vi "Lab Panel V5.10.vi"() -> ()   [LabVIEW 2013] (continued)
                            n848 = local write "data file error"(w1525) -> ()
                          }
                        }
                        n849 = Bundle(cluster=w1522, "STATUS"="STOP") -> (w1520:T4)  [unwired: 2 in]
                        n850 = local write "DISP LAB04-1"(w1520) -> ()
                      }
                    }
                  }
                  frame True {
                    n851 = local read "SIG LAB04-1"() -> (w1529:T2)
                    n852 = stacked-sequence {
                      seq-local: [w1540 _] -> [_ w1544]
                      tunnel: w1538 -> [_ w1554]
                      tunnel: w1537 -> [_ w1553]
                      tunnel: w1536 -> [_ w1552]
                      tunnel: w1535 -> [_ w1551]
                      tunnel: w1534 -> [_ w1550]
                      tunnel: [_ w1549] -> w1533
                      tunnel: w1532 -> [_ w1548]
                      tunnel: w1531 -> [_ w1547]
                      tunnel: w1530 -> [_ w1546]
                      tunnel: w1529 -> [w1539 w1545]
                      tunnel: w1528 -> [_ w1543]
                      frame #0 {
                        n853 = Unbundle(w1539) -> ("AMPS"=w1542:dbl)  [unwired: 4 out]
                        n854 = call "Check For Amps on v1.vi"("ID"="LAB04-1", "amps"=w1542) -> ("amps"=w1540:bool)  [unwired: 9 in]
                      }
                      frame #1 {
                        n855 = case shown="True" w1544 {
                          tunnel: w1554 -> [_ w1567]
                          tunnel: w1553 -> [_ w1566]
                          tunnel: w1552 -> [_ w1565]
                          tunnel: w1551 -> [_ w1564]
                          tunnel: w1550 -> [_ w1563]
                          tunnel: [errorcluster {"status"=FALSE, "code"=0, "source"=""} ("error out") w1562] -> w1549
                          tunnel: w1548 -> [_ w1561]
                          tunnel: w1547 -> [_ w1560]
                          tunnel: w1546 -> [_ w1559]
                          tunnel: w1545 -> [_ w1558]
                          tunnel: w1543 -> [_ w1557]
                          frame False {
                            w1555 = FALSE
                            n856 = local write "RUN LAB04-1"(w1555) -> ()
                            n857 = local write "run lab04-1"(w1555) -> ()
                          }
                          frame True {
                            n858 = stacked-sequence {
                              seq-local: [w1568 _ _ _ _] -> [_ w1592 _ _ _]
                              tunnel: w1567 -> [w1573 _ _ _ _]
                              tunnel: w1566 -> [w1569 _ _ _ _]
                              tunnel: w1565 -> [w1583 _ _ _ _]
                              tunnel: w1564 -> [w1576 _ _ _ _]
                              tunnel: w1563 -> [w1571 _ _ _ _]
                              tunnel: [_ w1587 _ _ _] -> w1562
                              tunnel: w1561 -> [_ _ _ w1613 _]
                              tunnel: w1560 -> [_ _ _ w1612 _]
                              tunnel: w1559 -> [_ _ _ w1611 _]
                              tunnel: w1558 -> [_ _ _ _ _]
                              tunnel: w1557 -> [_ _ _ _ w1627]
                              frame #0 {
                                w1570 = "\\"
                                n859 = local read "SET LAB04-1"() -> (w1578:T5)
                                n860 = case shown="\"CYCLE TEST\"" w1583 {
                                tunnel: ["L04-1-CHART TEST-" "L04-1-CYCLE TEST-" "L04-1-T-RISE TEST-"] -> w1579
                                frame "CHART TEST", Default {
                                }
                                frame "CYCLE TEST" {
                                }
                                frame "T-RISE TEST" {
                                }
                                }
                                n861 = Unbundle(w1578) -> ("DESCRIPTION"=w1577:string)  [unwired: 4 out]
                                n862 = Concatenate Strings(w1573, "\\", w1571, w1570, w1569, w1570) -> (w1580:string)
                                n863 = String To Path(string=w1580) -> (path=w1582:path)
                                n864 = Concatenate Strings(w1580, w1579, w1577, "-", w1576, ".tdms") -> (w1568:string)
                                n865 = Create Folder(path (use dialog)=w1582) -> (error out=w1581:errorcluster)  [unwired: 2 in, 2 out]
                                n866 = global write "Global 1.vi" "LAB04-1 FILE"(w1568) -> ()
                                n867 = call <vilib>:"Clear Errors.vi"("error in (no error)"=w1581) -> ()  [unwired: 6 in, 1 out]
                              }
                              frame #1 {
                                (unwired) FALSE
                                n868 = String To Path(string=w1592) -> (path=w1588:path)
                                n869 = TDMS Open(6:FALSE, 10:T20."create or replace" ("operation (0:open)"), 11:w1588) -> (0:w1587:errorcluster, 3:→"TDMS LAB04-1":refnum<k34>)  [unwired: 4 in]
                              }
                              frame #2 {
                                n870 = local read "SET LAB04-1"() -> (w1598:T5)
                                n871 = local read "TDMS LAB04-1"() -> (w1609:refnum<k34>)
                                n872 = Build Array("Testers Name", "Description", "Set Test Cycles", "T-Rise minutes", "T-Rise Deg C") -> (w1599:string[])
                                n873 = Unbundle(w1598) -> ("NAME"=w1597:string, "DESCRIPTION"=w1596:string, "CYCLES"=w1595:dbl, "T-RISE mins"=w1594:dbl, "T-RISE deg C"=w1593:dbl)
                                n874 = Number To Decimal String(number=w1595) -> (decimal integer string=w1608:string)  [unwired: 1 in]
                                n875 = Number To Decimal String(number=w1594) -> (decimal integer string=w1607:string)  [unwired: 1 in]
                                n876 = Number To Decimal String(number=w1593) -> (decimal integer string=w1606:string)  [unwired: 1 in]
                                n877 = Build Array(w1597, w1596, w1608, w1607, w1606) -> (w1605:string[])
                                n878 = TDMS Set Properties(5:w1605, 7:w1599, 11:w1609) -> ()  [unwired: 3 in, 4 out]
                              }
                              frame #3 {
                                n879 = local read "DISP LAB04-1"() -> (w1614:T4)
                                n880 = Concatenate Strings("LAB04-1  ", w1613) -> (w1615:string)
                                n881 = Two Button Dialog(message=w1615, 1:w1611, 2:w1612) -> (T button?=w1617:bool)
                                n882 = case shown="True" w1617 {
                                tunnel: w1614 -> [w1624 w1625]
                                tunnel: [w1624 w1625] -> w1621
                                tunnel: [w1623 w1626] -> w1620
                                tunnel: [w1622 w1626] -> w1619
                                frame False {
                                n883 = Unbundle(w1624) -> ("CYCLE"=w1623:dbl, "MINS"=w1622:dbl)  [unwired: 1 out]
                                }
                                frame True {
                                w1626 = 0.0
                                }
                                }
                                n884 = Bundle(cluster=w1621, "CYCLE"=w1620, "MINS"=w1619, "STATUS"="RUN") -> (w1610:T4)
                                n885 = local write "DISP LAB04-1"(w1610) -> ()
                              }
                              frame #4 {
                                n886 = local read "TEMP START LAB04-1"() -> (w1629:cluster{"TL":dbl, "TN":dbl})
                                n887 = Bundle(cluster=w1629, "TL"=w1627, "TN"=w1627) -> (w1628:cluster{"TL":dbl, "TN":dbl})
                                n888 = local write "TEMP START LAB04-1"(w1628) -> ()
                              }
                            }
                          }
                        }
                      }
                    }
                  }
                }
              }
              event "RUN LAB04-2": Value Change {
                n889 = event-data() -> ("NewVal"=w1634:bool)  [unwired: 1 in, 5 out]
                n890 = local write "run lab04-2"(w1634) -> ()
                n891 = case shown="True" w1634 {
                  tunnel: w1640 -> [_ w1678]
                  tunnel: w1639 -> [_ w1677]
                  tunnel: w1637 -> [w1642 w1676]
                  tunnel: w1638 -> [_ w1675]
                  tunnel: w1636 -> [_ w1674]
                  tunnel: [w1641 w1673] -> w1635
                  tunnel: w1633 -> [_ w1672]
                  tunnel: w1632 -> [_ w1671]
                  tunnel: w1631 -> [_ w1670]
                  tunnel: w1630 -> [_ w1668]
                  frame False {
                    # "stop test"
                    n892 = stacked-sequence {
                      tunnel: w1642 -> [w1651 _]
                      tunnel: [w1643 _] -> w1641
                      frame #0 {
                        n893 = local read "DISP LAB04-2"() -> (w1650:T4)
                        n894 = Unbundle(w1650) -> ("CYCLE"=w1648:dbl, "MINS"=w1649:dbl)  [unwired: 1 out]
                        n895 = case shown="\"CYCLE TEST\"" w1651 {
                          tunnel: w1649 -> [_ _ w1658]
                          tunnel: w1648 -> [w1656 w1657 _]
                          tunnel: [w1656 w1657 w1658] -> w1647
                          frame "CHART TEST", Default {
                          }
                          frame "CYCLE TEST" {
                          }
                          frame "T-RISE TEST" {
                          }
                        }
                        n896 = local read "TDMS LAB04-2"() -> (w1655:refnum<k34>)
                        n897 = Build Array("STOPPED") -> (w1652:string[])
                        n898 = Build Array(w1647) -> (w1646:dbl[])
                        n899 = TDMS Write(0:w1655, 5:"TEST RESULT", 7:w1652, 9:w1646) -> (4:w1644:refnum<k34>, 15:w1645:errorcluster)  [unwired: 2 in, 2 out]
                        n900 = TDMS Close(8:w1645, 11:w1644) -> (0:w1643:errorcluster)  [unwired: 1 out]
                      }
                      frame #1 {
                        n901 = local read "DISP LAB04-2"() -> (w1662:T4)
                        n902 = stacked-sequence {
                          tunnel: "LAB04-2" -> [w1664 w1666]
                          frame #0 {
                            n903 = call "sub vi - defrag tdms v1.vi"("panel id"=w1664) -> ("error out"=w1663:errorcluster)  [unwired: 10 in]
                            n904 = local write "data file error"(w1663) -> ()
                          }
                          frame #1 {
                            n905 = call "Save data file (stop) v3.vi"("panel id"=w1666) -> ("network file save error"=w1665:errorcluster)  [unwired: 9 in, 1 out]
                            n906 = local write "RESULT LAB04-2"(FALSE) -> ()
                            n907 = local write "data file error"(w1665) -> ()
                          }
                        }
                        n908 = Bundle(cluster=w1662, "STATUS"="STOP") -> (w1660:T4)  [unwired: 2 in]
                        n909 = local write "DISP LAB04-2"(w1660) -> ()
                      }
                    }
                  }
                  frame True {
                    n910 = local read "SIG LAB04-2"() -> (w1669:T2)
                    n911 = stacked-sequence {
                      seq-local: [w1680 _] -> [_ w1684]
                      tunnel: w1678 -> [_ w1694]
                      tunnel: w1677 -> [_ w1693]
                      tunnel: w1676 -> [_ w1692]
                      tunnel: w1675 -> [_ w1691]
                      tunnel: w1674 -> [_ w1690]
                      tunnel: [_ w1689] -> w1673
                      tunnel: w1672 -> [_ w1688]
                      tunnel: w1671 -> [_ w1687]
                      tunnel: w1670 -> [_ w1686]
                      tunnel: w1669 -> [w1679 w1685]
                      tunnel: w1668 -> [_ w1683]
                      frame #0 {
                        n912 = Unbundle(w1679) -> ("AMPS"=w1682:dbl)  [unwired: 4 out]
                        n913 = call "Check For Amps on v1.vi"("ID"="LAB04-2", "amps"=w1682) -> ("amps"=w1680:bool)  [unwired: 9 in]
                      }
                      frame #1 {
                        n914 = case shown="True" w1684 {
                          tunnel: w1694 -> [_ w1707]
                          tunnel: w1693 -> [_ w1706]
                          tunnel: w1692 -> [_ w1705]
                          tunnel: w1691 -> [_ w1704]
                          tunnel: w1690 -> [_ w1703]
                          tunnel: [errorcluster {"status"=FALSE, "code"=0, "source"=""} ("error out") w1702] -> w1689
                          tunnel: w1688 -> [_ w1701]
                          tunnel: w1687 -> [_ w1700]
                          tunnel: w1686 -> [_ w1699]
                          tunnel: w1685 -> [_ w1698]
                          tunnel: w1683 -> [_ w1697]
                          frame False {
                            w1695 = FALSE
                            n915 = local write "RUN LAB04-2"(w1695) -> ()
                            n916 = local write "run lab04-2"(w1695) -> ()
                          }
                          frame True {
                            n917 = stacked-sequence {
                              seq-local: [w1708 _ _ _ _] -> [_ w1732 _ _ _]
                              tunnel: w1707 -> [w1713 _ _ _ _]
                              tunnel: w1706 -> [w1709 _ _ _ _]
                              tunnel: w1705 -> [w1723 _ _ _ _]
                              tunnel: w1704 -> [w1716 _ _ _ _]
                              tunnel: w1703 -> [w1711 _ _ _ _]
                              tunnel: [_ w1727 _ _ _] -> w1702
                              tunnel: w1701 -> [_ _ _ w1753 _]
                              tunnel: w1700 -> [_ _ _ w1752 _]
                              tunnel: w1699 -> [_ _ _ w1751 _]
                              tunnel: w1698 -> [_ _ _ _ _]
                              tunnel: w1697 -> [_ _ _ _ w1767]
                              frame #0 {
                                w1710 = "\\"
                                n918 = local read "SET LAB04-2"() -> (w1718:T5)
                                n919 = case shown="\"CHART TEST\", Default" w1723 {
                                tunnel: ["L04-2-CHART TEST-" "L04-2-CYCLE TEST-" "L04-2-T-RISE TEST-"] -> w1719
                                frame "CHART TEST", Default {
                                }
                                frame "CYCLE TEST" {
                                }
                                frame "T-RISE TEST" {
                                }
                                }
                                n920 = Unbundle(w1718) -> ("DESCRIPTION"=w1717:string)  [unwired: 4 out]
                                n921 = Concatenate Strings(w1713, "\\", w1711, w1710, w1709, w1710) -> (w1720:string)
                                n922 = String To Path(string=w1720) -> (path=w1722:path)
                                n923 = Concatenate Strings(w1720, w1719, w1717, "-", w1716, ".tdms") -> (w1708:string)
                                n924 = Create Folder(path (use dialog)=w1722) -> (error out=w1721:errorcluster)  [unwired: 2 in, 2 out]
                                n925 = global write "Global 1.vi" "LAB04-2 FILE"(w1708) -> ()
                                n926 = call <vilib>:"Clear Errors.vi"("error in (no error)"=w1721) -> ()  [unwired: 6 in, 1 out]
                              }
                              frame #1 {
                                (unwired) FALSE
                                n927 = String To Path(string=w1732) -> (path=w1728:path)
                                n928 = TDMS Open(6:FALSE, 10:T20."create or replace" ("operation (0:open)"), 11:w1728) -> (0:w1727:errorcluster, 3:→"TDMS LAB04-2":refnum<k34>)  [unwired: 4 in]
                              }
                              frame #2 {
                                n929 = local read "SET LAB04-2"() -> (w1738:T5)
                                n930 = local read "TDMS LAB04-2"() -> (w1749:refnum<k34>)
                                n931 = Build Array("Testers Name", "Description", "Set Test Cycles", "T-Rise minutes", "T-Rise Deg C") -> (w1739:string[])
                                n932 = Unbundle(w1738) -> ("NAME"=w1737:string, "DESCRIPTION"=w1736:string, "CYCLES"=w1735:dbl, "T-RISE mins"=w1734:dbl, "T-RISE deg C"=w1733:dbl)
                                n933 = Number To Decimal String(number=w1735) -> (decimal integer string=w1748:string)  [unwired: 1 in]
                                n934 = Number To Decimal String(number=w1734) -> (decimal integer string=w1747:string)  [unwired: 1 in]
                                n935 = Number To Decimal String(number=w1733) -> (decimal integer string=w1746:string)  [unwired: 1 in]
                                n936 = Build Array(w1737, w1736, w1748, w1747, w1746) -> (w1745:string[])
                                n937 = TDMS Set Properties(5:w1745, 7:w1739, 11:w1749) -> ()  [unwired: 3 in, 4 out]
                              }
                              frame #3 {
                                n938 = local read "DISP LAB04-2"() -> (w1754:T4)
                                n939 = Concatenate Strings("LAB04-2 ", w1753) -> (w1755:string)
                                n940 = Two Button Dialog(message=w1755, 1:w1751, 2:w1752) -> (T button?=w1757:bool)
                                n941 = case shown="True" w1757 {
                                tunnel: w1754 -> [w1764 w1765]
                                tunnel: [w1764 w1765] -> w1761
                                tunnel: [w1763 w1766] -> w1760
                                tunnel: [w1762 w1766] -> w1759
                                frame False {
                                n942 = Unbundle(w1764) -> ("CYCLE"=w1763:dbl, "MINS"=w1762:dbl)  [unwired: 1 out]
                                }
                                frame True {
                                w1766 = 0.0
                                }
                                }
                                n943 = Bundle(cluster=w1761, "CYCLE"=w1760, "MINS"=w1759, "STATUS"="RUN") -> (w1750:T4)
                                n944 = local write "DISP LAB04-2"(w1750) -> ()
                              }
                              frame #4 {
                                n945 = local read "TEMP START LAB04-2"() -> (w1769:cluster{"TL":dbl, "TN":dbl})
                                n946 = Bundle(cluster=w1769, "TL"=w1767, "TN"=w1767) -> (w1768:cluster{"TL":dbl, "TN":dbl})
                                n947 = local write "TEMP START LAB04-2"(w1768) -> ()
                              }
                            }
                          }
                        }
                      }
                    }
                  }
                }
              }
              event "RUN LAB05-1": Value Change {
                n948 = event-data() -> ("NewVal"=w1774:bool)  [unwired: 1 in, 5 out]
                n949 = local write "run lab05-1"(w1774) -> ()
                n950 = case shown="True" w1774 {
                  tunnel: w1780 -> [_ w1818]
                  tunnel: w1779 -> [_ w1817]
                  tunnel: w1777 -> [w1782 w1816]
                  tunnel: w1778 -> [_ w1815]
                  tunnel: w1776 -> [_ w1814]
                  tunnel: [w1781 w1813] -> w1775
                  tunnel: w1773 -> [_ w1812]
                  tunnel: w1772 -> [_ w1811]
                  tunnel: w1771 -> [_ w1810]
                  tunnel: w1770 -> [_ w1808]
                  frame False {
                    # "stop test"
                    n951 = stacked-sequence {
                      tunnel: w1782 -> [w1791 _]
                      tunnel: [w1783 _] -> w1781
                      frame #0 {
                        n952 = local read "DISP LAB05-1"() -> (w1790:T4)
                        n953 = Unbundle(w1790) -> ("CYCLE"=w1788:dbl, "MINS"=w1789:dbl)  [unwired: 1 out]
                        n954 = case shown="\"CYCLE TEST\"" w1791 {
                          tunnel: w1789 -> [_ _ w1798]
                          tunnel: w1788 -> [w1796 w1797 _]
                          tunnel: [w1796 w1797 w1798] -> w1787
                          frame "CHART TEST", Default {
                          }
                          frame "CYCLE TEST" {
                          }
                          frame "T-RISE TEST" {
                          }
                        }
                        n955 = local read "TDMS LAB05-1"() -> (w1795:refnum<k34>)
                        n956 = Build Array("STOPPED") -> (w1792:string[])
                        n957 = Build Array(w1787) -> (w1786:dbl[])
                        n958 = TDMS Write(0:w1795, 5:"TEST RESULT", 7:w1792, 9:w1786) -> (4:w1784:refnum<k34>, 15:w1785:errorcluster)  [unwired: 2 in, 2 out]
                        n959 = TDMS Close(8:w1785, 11:w1784) -> (0:w1783:errorcluster)  [unwired: 1 out]
                      }
                      frame #1 {
                        n960 = local read "DISP LAB05-1"() -> (w1802:T4)
                        n961 = stacked-sequence {
                          tunnel: "LAB05-1" -> [w1804 w1806]
                          frame #0 {
                            n962 = call "sub vi - defrag tdms v1.vi"("panel id"=w1804) -> ("error out"=w1803:errorcluster)  [unwired: 10 in]
                            n963 = local write "data file error"(w1803) -> ()
                          }
                          frame #1 {
                            n964 = call "Save data file (stop) v3.vi"("panel id"=w1806) -> ("network file save error"=w1805:errorcluster)  [unwired: 9 in, 1 out]
                            n965 = local write "RESULT LAB05-1"(FALSE) -> ()
                            n966 = local write "data file error"(w1805) -> ()
                          }
                        }
                        n967 = Bundle(cluster=w1802, "STATUS"="STOP") -> (w1800:T4)  [unwired: 2 in]
                        n968 = local write "DISP LAB05-1"(w1800) -> ()
                      }
                    }
                  }
                  frame True {
                    n969 = local read "SIG LAB05-1"() -> (w1809:T2)
                    n970 = stacked-sequence {
                      seq-local: [w1820 _] -> [_ w1824]
                      tunnel: w1818 -> [_ w1834]
                      tunnel: w1817 -> [_ w1833]
                      tunnel: w1816 -> [_ w1832]
                      tunnel: w1815 -> [_ w1831]
                      tunnel: w1814 -> [_ w1830]
                      tunnel: [_ w1829] -> w1813
                      tunnel: w1812 -> [_ w1828]
                      tunnel: w1811 -> [_ w1827]
                      tunnel: w1810 -> [_ w1826]
                      tunnel: w1809 -> [w1819 w1825]
                      tunnel: w1808 -> [_ w1823]
                      frame #0 {
                        n971 = Unbundle(w1819) -> ("AMPS"=w1822:dbl)  [unwired: 4 out]
                        n972 = call "Check For Amps on v1.vi"("ID"="LAB05-1", "amps"=w1822) -> ("amps"=w1820:bool)  [unwired: 9 in]
                      }
                      frame #1 {
                        n973 = case shown="True" w1824 {
                          tunnel: w1834 -> [_ w1847]
                          tunnel: w1833 -> [_ w1846]
                          tunnel: w1832 -> [_ w1845]
                          tunnel: w1831 -> [_ w1844]
                          tunnel: w1830 -> [_ w1843]
                          tunnel: [errorcluster {"status"=FALSE, "code"=0, "source"=""} ("error out") w1842] -> w1829
                          tunnel: w1828 -> [_ w1841]
                          tunnel: w1827 -> [_ w1840]
                          tunnel: w1826 -> [_ w1839]
                          tunnel: w1825 -> [_ w1838]
                          tunnel: w1823 -> [_ w1837]
                          frame False {
                            w1835 = FALSE
                            n974 = local write "RUN LAB05-1"(w1835) -> ()
                            n975 = local write "run lab05-1"(w1835) -> ()
                          }
                          frame True {
                            n976 = stacked-sequence {
                              seq-local: [w1848 _ _ _ _] -> [_ w1872 _ _ _]
                              tunnel: w1847 -> [w1853 _ _ _ _]
                              tunnel: w1846 -> [w1849 _ _ _ _]
                              tunnel: w1845 -> [w1863 _ _ _ _]
                              tunnel: w1844 -> [w1856 _ _ _ _]
                              tunnel: w1843 -> [w1851 _ _ _ _]
                              tunnel: [_ w1867 _ _ _] -> w1842
                              tunnel: w1841 -> [_ _ _ w1892 _]
                              tunnel: w1840 -> [_ _ _ w1891 _]
                              tunnel: w1839 -> [_ _ _ w1890 _]
                              tunnel: w1838 -> [_ _ _ _ _]
                              tunnel: w1837 -> [_ _ _ _ w1907]
                              frame #0 {
                                w1850 = "\\"
                                n977 = local read "SET LAB05-1"() -> (w1858:T5)
                                n978 = case shown="\"CYCLE TEST\"" w1863 {
                                tunnel: ["L05-1-CHART TEST-" "L05-1-CYCLE TEST-" "L05-1-T-RISE TEST-"] -> w1859
                                frame "CHART TEST", Default {
                                }
                                frame "CYCLE TEST" {
                                }
                                frame "T-RISE TEST" {
                                }
                                }
                                n979 = Unbundle(w1858) -> ("DESCRIPTION"=w1857:string)  [unwired: 4 out]
                                n980 = Concatenate Strings(w1853, "\\", w1851, w1850, w1849, w1850) -> (w1860:string)
                                n981 = String To Path(string=w1860) -> (path=w1862:path)
                                n982 = Concatenate Strings(w1860, w1859, w1857, "-", w1856, ".tdms") -> (w1848:string)
                                n983 = Create Folder(path (use dialog)=w1862) -> (error out=w1861:errorcluster)  [unwired: 2 in, 2 out]
                                n984 = global write "Global 1.vi" "LAB05-1 FILE"(w1848) -> ()
                                n985 = call <vilib>:"Clear Errors.vi"("error in (no error)"=w1861) -> ()  [unwired: 6 in, 1 out]
                              }
                              frame #1 {
                                (unwired) FALSE
                                n986 = String To Path(string=w1872) -> (path=w1868:path)
                                n987 = TDMS Open(6:FALSE, 10:T20."create or replace" ("operation (0:open)"), 11:w1868) -> (0:w1867:errorcluster, 3:→"TDMS LAB05-1":refnum<k34>)  [unwired: 4 in]
                              }
                              frame #2 {
                                n988 = local read "SET LAB05-1"() -> (w1878:T5)
                                n989 = local read "TDMS LAB05-1"() -> (w1889:refnum<k34>)
                                n990 = Build Array("Testers Name", "Description", "Set Test Cycles", "T-Rise minutes", "T-Rise Deg C") -> (w1879:string[])
                                n991 = Unbundle(w1878) -> ("NAME"=w1877:string, "DESCRIPTION"=w1876:string, "CYCLES"=w1875:dbl, "T-RISE mins"=w1874:dbl, "T-RISE deg C"=w1873:dbl)
                                n992 = Number To Decimal String(number=w1875) -> (decimal integer string=w1888:string)  [unwired: 1 in]
                                n993 = Number To Decimal String(number=w1874) -> (decimal integer string=w1887:string)  [unwired: 1 in]
                                n994 = Number To Decimal String(number=w1873) -> (decimal integer string=w1886:string)  [unwired: 1 in]
                                n995 = Build Array(w1877, w1876, w1888, w1887, w1886) -> (w1885:string[])
                                n996 = TDMS Set Properties(5:w1885, 7:w1879, 11:w1889) -> ()  [unwired: 3 in, 4 out]
                              }
                              frame #3 {
                                n997 = local read "DISP LAB05-1"() -> (w1894:T4)
                                n998 = Concatenate Strings("LAB05-1  ", w1892) -> (w1895:string)
                                n999 = Two Button Dialog(message=w1895, 1:w1890, 2:w1891) -> (T button?=w1897:bool)
                                n1000 = case shown="True" w1897 {
                                tunnel: w1894 -> [w1904 w1905]
                                tunnel: [w1904 w1905] -> w1901
                                tunnel: [w1903 w1906] -> w1900
                                tunnel: [w1902 w1906] -> w1899
                                frame False {
                                n1001 = Unbundle(w1904) -> ("CYCLE"=w1903:dbl, "MINS"=w1902:dbl)  [unwired: 1 out]
                                }
                                frame True {
                                w1906 = 0.0
                                }
                                }
                                n1002 = Bundle(cluster=w1901, "CYCLE"=w1900, "MINS"=w1899, "STATUS"="RUN") -> (w1893:T4)
                                n1003 = local write "DISP LAB05-1"(w1893) -> ()
                              }
                              frame #4 {
                                n1004 = local read "TEMP START LAB05-1"() -> (w1909:cluster{"TL":dbl, "TN":dbl})
                                n1005 = Bundle(cluster=w1909, "TL"=w1907, "TN"=w1907) -> (w1908:cluster{"TL":dbl, "TN":dbl})
                                n1006 = local write "TEMP START LAB05-1"(w1908) -> ()
                              }
                            }
                          }
                        }
                      }
                    }
                  }
                }
              }
              event "RUN LAB05-2": Value Change {
                n1007 = event-data() -> ("NewVal"=w1915:bool)  [unwired: 1 in, 5 out]
                n1008 = local read "SIG LAB05-2"() -> (w1911:T2)
                n1009 = case shown="True" w1915 {
                  tunnel: w1921 -> [_ w1959]
                  tunnel: w1920 -> [_ w1958]
                  tunnel: w1918 -> [w1923 w1957]
                  tunnel: w1919 -> [_ w1956]
                  tunnel: w1917 -> [_ w1955]
                  tunnel: [w1922 w1954] -> w1916
                  tunnel: w1914 -> [_ w1953]
                  tunnel: w1913 -> [_ w1952]
                  tunnel: w1912 -> [_ w1951]
                  tunnel: w1911 -> [_ w1950]
                  tunnel: w1910 -> [_ w1949]
                  frame False {
                    # "stop test"
                    n1010 = stacked-sequence {
                      tunnel: w1923 -> [w1932 _]
                      tunnel: [w1924 _] -> w1922
                      frame #0 {
                        n1011 = local read "DISP LAB05-2"() -> (w1931:T4)
                        n1012 = Unbundle(w1931) -> ("CYCLE"=w1929:dbl, "MINS"=w1930:dbl)  [unwired: 1 out]
                        n1013 = case shown="\"CYCLE TEST\"" w1932 {
                          tunnel: w1930 -> [_ _ w1939]
                          tunnel: w1929 -> [w1937 w1938 _]
                          tunnel: [w1937 w1938 w1939] -> w1928
                          frame "CHART TEST", Default {
                          }
                          frame "CYCLE TEST" {
                          }
                          frame "T-RISE TEST" {
                          }
                        }
                        n1014 = local read "TDMS LAB05-2"() -> (w1936:refnum<k34>)
                        n1015 = Build Array("STOPPED") -> (w1933:string[])
                        n1016 = Build Array(w1928) -> (w1927:dbl[])
                        n1017 = TDMS Write(0:w1936, 5:"TEST RESULT", 7:w1933, 9:w1927) -> (4:w1925:refnum<k34>, 15:w1926:errorcluster)  [unwired: 2 in, 2 out]
                        n1018 = TDMS Close(8:w1926, 11:w1925) -> (0:w1924:errorcluster)  [unwired: 1 out]
                      }
                      frame #1 {
                        n1019 = local read "DISP LAB05-2"() -> (w1943:T4)
                        n1020 = stacked-sequence {
                          tunnel: "LAB05-2" -> [w1945 w1947]
                          frame #0 {
                            n1021 = call "sub vi - defrag tdms v1.vi"("panel id"=w1945) -> ("error out"=w1944:errorcluster)  [unwired: 10 in]
                            n1022 = local write "data file error"(w1944) -> ()
                          }
                          frame #1 {
                            n1023 = local write "RESULT LAB05-2"(FALSE) -> ()
                            n1024 = call "Save data file (stop) v3.vi"("panel id"=w1947) -> ("network file save error"=w1946:errorcluster)  [unwired: 9 in, 1 out]
                            n1025 = local write "data file error"(w1946) -> ()
                          }
                        }
                        n1026 = Bundle(cluster=w1943, "STATUS"="STOP") -> (w1941:T4)  [unwired: 2 in]
                        n1027 = local write "DISP LAB05-2"(w1941) -> ()
                      }
                    }
                  }
                  frame True {
                    n1028 = stacked-sequence {
                      seq-local: [w1961 _] -> [_ w1965]
                      tunnel: w1959 -> [_ w1975]
                      tunnel: w1958 -> [_ w1974]
                      tunnel: w1957 -> [_ w1973]
                      tunnel: w1956 -> [_ w1972]
                      tunnel: w1955 -> [_ w1971]
                      tunnel: [_ w1970] -> w1954
                      tunnel: w1953 -> [_ w1969]
                      tunnel: w1952 -> [_ w1968]
                      tunnel: w1951 -> [_ w1967]
                      tunnel: w1950 -> [w1960 w1966]
                      tunnel: w1949 -> [_ w1964]
                      frame #0 {
                        n1029 = Unbundle(w1960) -> ("AMPS"=w1963:dbl)  [unwired: 4 out]
                        n1030 = call "Check For Amps on v1.vi"("ID"="LAB05-2", "amps"=w1963) -> ("amps"=w1961:bool)  [unwired: 9 in]
                      }
                      frame #1 {
                        n1031 = case shown="True" w1965 {
                          tunnel: w1975 -> [_ w1988]
                          tunnel: w1974 -> [_ w1987]
                          tunnel: w1973 -> [_ w1986]
                          tunnel: w1972 -> [_ w1985]
                          tunnel: w1971 -> [_ w1984]
                          tunnel: [errorcluster {"status"=FALSE, "code"=0, "source"=""} ("error out") w1983] -> w1970
                          tunnel: w1969 -> [_ w1982]
                          tunnel: w1968 -> [_ w1981]
                          tunnel: w1967 -> [_ w1980]
                          tunnel: w1966 -> [_ w1979]
                          tunnel: w1964 -> [_ w1978]
                          frame False {
                            w1976 = FALSE
                            n1032 = local write "RUN LAB05-2"(w1976) -> ()
                            n1033 = local write "run lab05-2"(w1976) -> ()
                          }
                          frame True {
                            n1034 = stacked-sequence {
                              seq-local: [w1989 _ _ _ _] -> [_ w2013 _ _ _]
                              tunnel: w1988 -> [w1994 _ _ _ _]
                              tunnel: w1987 -> [w1990 _ _ _ _]
                              tunnel: w1986 -> [w2004 _ _ _ _]
                              tunnel: w1985 -> [w1997 _ _ _ _]
                              tunnel: w1984 -> [w1992 _ _ _ _]
                              tunnel: [_ w2008 _ _ _] -> w1983
                              tunnel: w1982 -> [_ _ _ w2033 _]
                              tunnel: w1981 -> [_ _ _ w2032 _]
                              tunnel: w1980 -> [_ _ _ w2031 _]
                              tunnel: w1979 -> [_ _ _ _ _]
                              tunnel: w1978 -> [_ _ _ _ w2048]
                              frame #0 {
                                w1991 = "\\"
                                n1035 = local read "SET LAB05-2"() -> (w1999:T5)
                                n1036 = case shown="\"CYCLE TEST\"" w2004 {
                                tunnel: ["L05-2-CHART TEST-" "L05-2-CYCLE TEST-" "L05-2-T-RISE TEST-"] -> w2000
                                frame "CHART TEST", Default {
                                }
                                frame "CYCLE TEST" {
                                }
                                frame "T-RISE TEST" {
                                }
                                }
                                n1037 = Unbundle(w1999) -> ("DESCRIPTION"=w1998:string)  [unwired: 4 out]
                                n1038 = Concatenate Strings(w1994, "\\", w1992, w1991, w1990, w1991) -> (w2001:string)
                                n1039 = String To Path(string=w2001) -> (path=w2003:path)
                                n1040 = Concatenate Strings(w2001, w2000, w1998, "-", w1997, ".tdms") -> (w1989:string)
                                n1041 = Create Folder(path (use dialog)=w2003) -> (error out=w2002:errorcluster)  [unwired: 2 in, 2 out]
                                n1042 = global write "Global 1.vi" "LAB05-2 FILE"(w1989) -> ()
                                n1043 = call <vilib>:"Clear Errors.vi"("error in (no error)"=w2002) -> ()  [unwired: 6 in, 1 out]
                              }
                              frame #1 {
                                (unwired) FALSE
                                n1044 = String To Path(string=w2013) -> (path=w2009:path)
                                n1045 = TDMS Open(6:FALSE, 10:T20."create or replace" ("operation (0:open)"), 11:w2009) -> (0:w2008:errorcluster, 3:→"TDMS LAB05-2":refnum<k34>)  [unwired: 4 in]
                              }
                              frame #2 {
                                n1046 = local read "SET LAB05-2"() -> (w2019:T5)
                                n1047 = local read "TDMS LAB05-2"() -> (w2030:refnum<k34>)
                                n1048 = Build Array("Testers Name", "Description", "Set Test Cycles", "T-Rise minutes", "T-Rise Deg C") -> (w2020:string[])
                                n1049 = Unbundle(w2019) -> ("NAME"=w2018:string, "DESCRIPTION"=w2017:string, "CYCLES"=w2016:dbl, "T-RISE mins"=w2015:dbl, "T-RISE deg C"=w2014:dbl)
                                n1050 = Number To Decimal String(number=w2016) -> (decimal integer string=w2029:string)  [unwired: 1 in]
                                n1051 = Number To Decimal String(number=w2015) -> (decimal integer string=w2028:string)  [unwired: 1 in]
                                n1052 = Number To Decimal String(number=w2014) -> (decimal integer string=w2027:string)  [unwired: 1 in]
                                n1053 = Build Array(w2018, w2017, w2029, w2028, w2027) -> (w2026:string[])
                                n1054 = TDMS Set Properties(5:w2026, 7:w2020, 11:w2030) -> ()  [unwired: 3 in, 4 out]
                              }
                              frame #3 {
                                n1055 = local read "DISP LAB05-2"() -> (w2035:T4)
                                n1056 = Concatenate Strings("LAB05-2  ", w2033) -> (w2036:string)
                                n1057 = Two Button Dialog(message=w2036, 1:w2031, 2:w2032) -> (T button?=w2038:bool)
                                n1058 = case shown="True" w2038 {
                                tunnel: w2035 -> [w2045 w2046]
                                tunnel: [w2045 w2046] -> w2042
                                tunnel: [w2044 w2047] -> w2041
                                tunnel: [w2043 w2047] -> w2040
                                frame False {
                                n1059 = Unbundle(w2045) -> ("CYCLE"=w2044:dbl, "MINS"=w2043:dbl)  [unwired: 1 out]
                                }
                                frame True {
                                w2047 = 0.0
                                }
                                }
                                n1060 = Bundle(cluster=w2042, "CYCLE"=w2041, "MINS"=w2040, "STATUS"="RUN") -> (w2034:T4)
                                n1061 = local write "DISP LAB05-2"(w2034) -> ()
                              }
                              frame #4 {
                                n1062 = local read "TEMP START LAB05-2"() -> (w2050:cluster{"TL":dbl, "TN":dbl})
                                n1063 = Bundle(cluster=w2050, "TL"=w2048, "TN"=w2048) -> (w2049:cluster{"TL":dbl, "TN":dbl})
                                n1064 = local write "TEMP START LAB05-2"(w2049) -> ()
                              }
                            }
                          }
                        }
                      }
                    }
                  }
                }
                n1065 = local write "run lab05-2"(w1915) -> ()
              }
            }
            n1066 = local write "data file error"(w619) -> ()
          }
          frame #4 {
            # "check if test cycles reached for cycle tests, if so then test pass"
            n1067 = stacked-sequence {
              tunnel: w2070 -> [_ _ _ _ _ _ _ _ _ _]
              tunnel: w2069 -> [_ _ _ _ _ _ _ _ _ _]
              tunnel: w2068 -> [_ _ _ _ _ _ _ _ _ _]
              tunnel: w2067 -> [_ _ _ _ _ _ _ _ _ _]
              tunnel: w2066 -> [_ _ _ _ _ _ _ _ _ _]
              tunnel: w2065 -> [_ _ _ _ _ _ _ _ _ _]
              tunnel: w2064 -> [_ _ _ _ _ _ _ _ _ _]
              tunnel: w2063 -> [_ _ _ _ _ _ _ _ _ _]
              tunnel: w2062 -> [_ _ _ _ _ _ _ _ _ _]
              tunnel: w2061 -> [_ _ _ _ _ _ _ _ _ _]
              tunnel: w2060 -> [w2076 _ _ _ _ _ _ _ _ _]
              tunnel: w2059 -> [_ w2111 _ _ _ _ _ _ _ _]
              tunnel: w2058 -> [_ _ w2151 _ _ _ _ _ _ _]
              tunnel: w2057 -> [_ _ _ w2191 _ _ _ _ _ _]
              tunnel: w2056 -> [_ _ _ _ w2231 _ _ _ _ _]
              tunnel: w2055 -> [_ _ _ _ _ w2271 _ _ _ _]
              tunnel: w2054 -> [_ _ _ _ _ _ w2311 _ _ _]
              tunnel: w2053 -> [_ _ _ _ _ _ _ w2351 _ _]
              tunnel: w2052 -> [_ _ _ _ _ _ _ _ w2391 _]
              tunnel: w2051 -> [_ _ _ _ _ _ _ _ _ w2431]
              frame #0 {
                # "LAB01-1"
                n1068 = Less?(x=w2076, y=2) -> (x < y?=w2074:bool)
                n1069 = local read "DISP LAB01-1"() -> (w2077:T4)
                n1070 = Unbundle(w2077) -> ("STATUS"=w2071:string)  [unwired: 2 out]
                n1071 = Equal?(x=w2071, y="RUN") -> (x = y?=w2073:bool)
                n1072 = And(x=w2073, y=w2074) -> (x .and. y?=w2072:bool)
                n1073 = case shown="True" w2072 {
                  tunnel: w2077 -> [_ w2082]
                  tunnel: w2076 -> [_ w2086]
                  frame False {
                  }
                  frame True {
                    n1074 = local read "SET LAB01-1"() -> (w2088:T5)
                    n1075 = local read "TDMS LAB01-1"() -> (w2081:refnum<k34>)
                    n1076 = Unbundle(w2088) -> ("CYCLES"=w2079:dbl, "T-RISE mins"=w2085:dbl)  [unwired: 3 out]
                    n1077 = case shown="\"CYCLE TEST\"" w2086 {
                      tunnel: w2085 -> [_ _ w2095]
                      tunnel: [w2090 w2092 w2095] -> w2084
                      tunnel: w2079 -> [w2090 w2092 _]
                      tunnel: ["CHART PASS" "CYCLE PASS" "T-RISE PASS"] -> w2083
                      frame "CHART TEST", Default {
                      }
                      frame "CYCLE TEST" {
                      }
                      frame "T-RISE TEST" {
                      }
                    }
                    n1078 = Unbundle(w2082) -> ("CYCLE"=w2087:dbl)  [unwired: 2 out]
                    n1079 = Increment(x=w2079) -> (x+1=w2080:dbl)
                    n1080 = Greater Or Equal?(x=w2087, y=w2080) -> (x >= y?=w2089:bool)
                    n1081 = case shown="True" w2089 {
                      tunnel: w2084 -> [w2099 _]
                      tunnel: w2083 -> [w2098 _]
                      tunnel: w2082 -> [w2097 _]
                      tunnel: w2081 -> [w2096 _]
                      frame True {
                        n1082 = stacked-sequence {
                          tunnel: w2099 -> [w2103 _]
                          tunnel: w2098 -> [w2101 w2107]
                          tunnel: w2097 -> [_ w2110]
                          tunnel: w2096 -> [w2100 _]
                          frame #0 {
                            n1083 = Build Array(w2101) -> (w2104:string[])
                            n1084 = Build Array(w2103) -> (w2102:dbl[])
                            n1085 = TDMS Write(0:w2100, 5:"TEST PASS", 7:w2104, 9:w2102) -> (15:w2106:errorcluster)  [unwired: 2 in, 3 out]
                            n1086 = local write "data file error"(w2106) -> ()
                          }
                          frame #1 {
                            n1087 = Bundle(cluster=w2110, "STATUS"=w2107) -> (w2108:T4)  [unwired: 2 in]
                            n1088 = local write "RESULT LAB01-1"(TRUE) -> ()
                            n1089 = local write "DISP LAB01-1"(w2108) -> ()
                          }
                        }
                      }
                      frame False {
                      }
                    }
                  }
                }
              }
              frame #1 {
                # "LAB01-2"
                n1090 = Less?(x=w2111, y=2) -> (x < y?=w2114:bool)
                n1091 = local read "DISP LAB01-2"() -> (w2116:T4)
                n1092 = Unbundle(w2116) -> ("STATUS"=w2117:string)  [unwired: 2 out]
                n1093 = Equal?(x=w2117, y="RUN") -> (x = y?=w2113:bool)
                n1094 = And(x=w2113, y=w2114) -> (x .and. y?=w2112:bool)
                n1095 = case shown="True" w2112 {
                  tunnel: w2116 -> [_ w2122]
                  tunnel: w2111 -> [_ w2126]
                  frame False {
                  }
                  frame True {
                    n1096 = local read "SET LAB01-2"() -> (w2128:T5)
                    n1097 = local read "TDMS LAB01-2"() -> (w2121:refnum<k34>)
                    n1098 = Unbundle(w2128) -> ("CYCLES"=w2119:dbl, "T-RISE mins"=w2125:dbl)  [unwired: 3 out]
                    n1099 = case shown="\"T-RISE TEST\"" w2126 {
                      tunnel: w2125 -> [_ _ w2135]
                      tunnel: [w2130 w2132 w2135] -> w2124
                      tunnel: w2119 -> [w2130 w2132 _]
                      tunnel: ["CHART PASS" "CYCLE PASS" "T-RISE PASS"] -> w2123
                      frame "CHART TEST", Default {
                      }
                      frame "CYCLE TEST" {
                      }
                      frame "T-RISE TEST" {
                      }
                    }
                    n1100 = Unbundle(w2122) -> ("CYCLE"=w2127:dbl)  [unwired: 2 out]
                    n1101 = Increment(x=w2119) -> (x+1=w2120:dbl)
                    n1102 = Greater Or Equal?(x=w2127, y=w2120) -> (x >= y?=w2129:bool)
                    n1103 = case shown="True" w2129 {
                      tunnel: w2124 -> [w2139 _]
                      tunnel: w2123 -> [w2138 _]
                      tunnel: w2122 -> [w2137 _]
                      tunnel: w2121 -> [w2136 _]
                      frame True {
                        n1104 = stacked-sequence {
                          tunnel: w2139 -> [w2143 _]
                          tunnel: w2138 -> [w2141 w2147]
                          tunnel: w2137 -> [_ w2150]
                          tunnel: w2136 -> [w2140 _]
                          frame #0 {
                            n1105 = Build Array(w2141) -> (w2144:string[])
                            n1106 = Build Array(w2143) -> (w2142:dbl[])
                            n1107 = TDMS Write(0:w2140, 5:"TEST PASS", 7:w2144, 9:w2142) -> (15:w2146:errorcluster)  [unwired: 2 in, 3 out]
                            n1108 = local write "data file error"(w2146) -> ()
                          }
                          frame #1 {
                            n1109 = Bundle(cluster=w2150, "STATUS"=w2147) -> (w2148:T4)  [unwired: 2 in]
                            n1110 = local write "RESULT LAB01-2"(TRUE) -> ()
                            n1111 = local write "DISP LAB01-2"(w2148) -> ()
                          }
                        }
                      }
                      frame False {
                      }
                    }
                  }
                }
              }
              frame #2 {
                # "LAB02-1"
                n1112 = Less?(x=w2151, y=2) -> (x < y?=w2154:bool)
                n1113 = local read "DISP LAB02-1"() -> (w2156:T4)
                n1114 = Unbundle(w2156) -> ("STATUS"=w2157:string)  [unwired: 2 out]
                n1115 = Equal?(x=w2157, y="RUN") -> (x = y?=w2153:bool)
                n1116 = And(x=w2153, y=w2154) -> (x .and. y?=w2152:bool)
                n1117 = case shown="True" w2152 {
                  tunnel: w2156 -> [_ w2162]
                  tunnel: w2151 -> [_ w2166]
                  frame False {
                  }
                  frame True {
                    n1118 = local read "SET LAB02-1"() -> (w2168:T5)
                    n1119 = local read "TDMS LAB02-1"() -> (w2161:refnum<k34>)
                    n1120 = Unbundle(w2162) -> ("CYCLE"=w2167:dbl)  [unwired: 2 out]
                    n1121 = Unbundle(w2168) -> ("CYCLES"=w2159:dbl, "T-RISE mins"=w2165:dbl)  [unwired: 3 out]
                    n1122 = case shown="\"T-RISE TEST\"" w2166 {
                      tunnel: w2165 -> [_ _ w2175]
                      tunnel: [w2170 w2172 w2175] -> w2164
